vi "Insert Report.vi"(8 "error in (no error)":errorcluster, 10 "?":T1, 11 "Path":path) -> (0 "error out":errorcluster)   [LabVIEW 2017]
uses:
  Controls/Testscreen_Input cluster.ctl
  <vilib>/addons/database/Connection.llb/Conn ObjectReference.ctl
  <vilib>/addons/database/NI_Database_API.lvlib
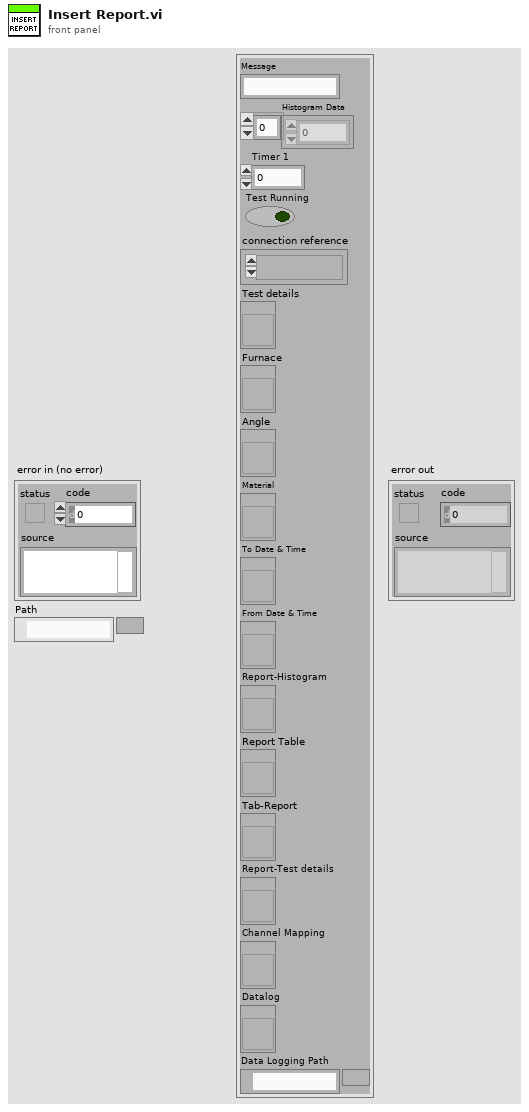
[diagram p1: front panel]
types:
  T1 = typedef "Testscreen_Input cluster.ctl" = cluster{"Message":string, "Histogram Data":i32[], "Timer 1":u32, "Test Running":bool, "connection reference":T2, "Test details":refnum<vi>, "Furnace":refnum<vi>, "Angle":refnum<vi>, "Material":refnum<vi>, "To Date & Time":refnum<vi>, "From Date & Time":refnum<vi>, "Report-Histogram":refnum<vi>, "Report Table":refnum<vi>, "Tab-Report":refnum<vi>, "Report-Test details":refnum<vi>, "Channel Mapping":refnum<vi>, "Datalog":refnum<vi>, "Data Logging Path":path}
  T2 = typedef "NI_Database_API.lvlib/Conn ObjectReference.ctl" = refnum<k1>
  T3 = cluster{"ID":string, "Test Name":string, "Flowrate":string, "Furnace":string, "Material":string, "Angle":string, "Tested By":string}
  T4 = cluster{i32, "date/time string":string, dbl, string, "ID":string, "Test Name":string, "Tested By":string, "Flowrate":string, "Furnace":string, "Material":string, "Angle":string}
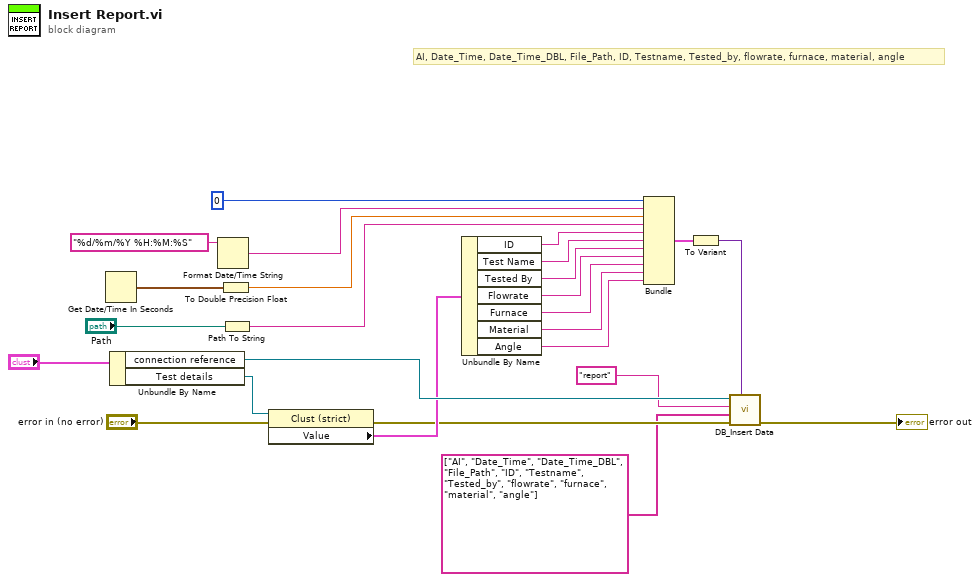
[diagram p0: block diagram]
diagram:
  # "AI, Date_Time, Date_Time_DBL, File_Path, ID, Testname, Tested_by, flowrate, furnace, material, angle"
  n1 = Get Date/Time In Seconds() -> (seconds since 1Jan1904=w22:timestamp)
  n2 = Unbundle By Name("?") -> ("connection reference"=w16:T2, "Test details"=w15:refnum<vi>)
  n3 = Format Date/Time String(time format string (%c)="%d/%m/%Y %H:%M:%S") -> (date/time string=w23:string)  [unwired: 2 in]
  n4 = To Double Precision Float(number=w22) -> (double precision float=w21:dbl)
  n5 = Path To String(path="Path") -> (string=w19:string)
  n6 = property class="Clust (strict)"(reference=w15, error in="error in (no error)") -> (error out=w12:errorcluster, "Value"=w14:T3)  [unwired: 1 out]
  n7 = Unbundle By Name(w14) -> ("ID"=w11:string, "Test Name"=w10:string, "Tested By"=w9:string, "Flowrate"=w8:string, "Furnace"=w7:string, "Material"=w6:string, "Angle"=w5:string)
  n8 = Bundle(0, "date/time string"=w23, w21, w19, "ID"=w11, "Test Name"=w10, "Tested By"=w9, "Flowrate"=w8, "Furnace"=w7, "Material"=w6, "Angle"=w5) -> (w17:T4)  [unwired: 1 in]
  n9 = To Variant(anything=w17) -> (Variant=w2:variant)
  n10 = call "DB_Insert Data.vi"("data"=w2, "error in (no error)"=w12, "columns"=string[] ["AI", "Date_Time", "Date_Time_DBL", "File_Path", "ID", "Testname", "Tested_by", "flowrate", "furnace", "material", "angle"], "table"="report", "connection reference"=w16) -> ("error out"=→"error out":errorcluster)  [unwired: 6 in]
